vi "ccd_triggeredacquire_bkup.vi"() -> ()   [LabVIEW 2009]
panel:
  out "output path":path
  out "Y 3":dbl
  out "X 3":dbl
  out "Y 2":dbl
  out "X 2":dbl
  out "Image 2":T1(plugin-control)
  out "Image":T1(plugin-control)
  out "cameraName":dbl
  out "imageType":dbl
  out "trigger_number":dbl
  out "framenumber":dbl
  out "Y":dbl
  out "X":dbl
  in  "Trigger action":u32(ring)=1 items=["Disabled", "Trigger start of acquisition", "Trigger start of each buffer list", "Trigger each buffer", "Trigger each line (linescan)", "Trigger end of acquisition"]
  in  "Trigger Type":u32(ring) items=["External", "RTSI", "ISO In"]
  in  "Data frames / trigger":dbl=10.0
  in  "Video Frames / Data frame":dbl=15.0
  in  "GO":bool
  in  "stop":bool
  in  "Manual (up) or automatic (down)":bool
  in  "Or, read path automatically from:":path=path "\\\\Foghorn.bio.brandeis.edu\\remote"
  in  "Manual save directory":string
  in  "Manual save path":path
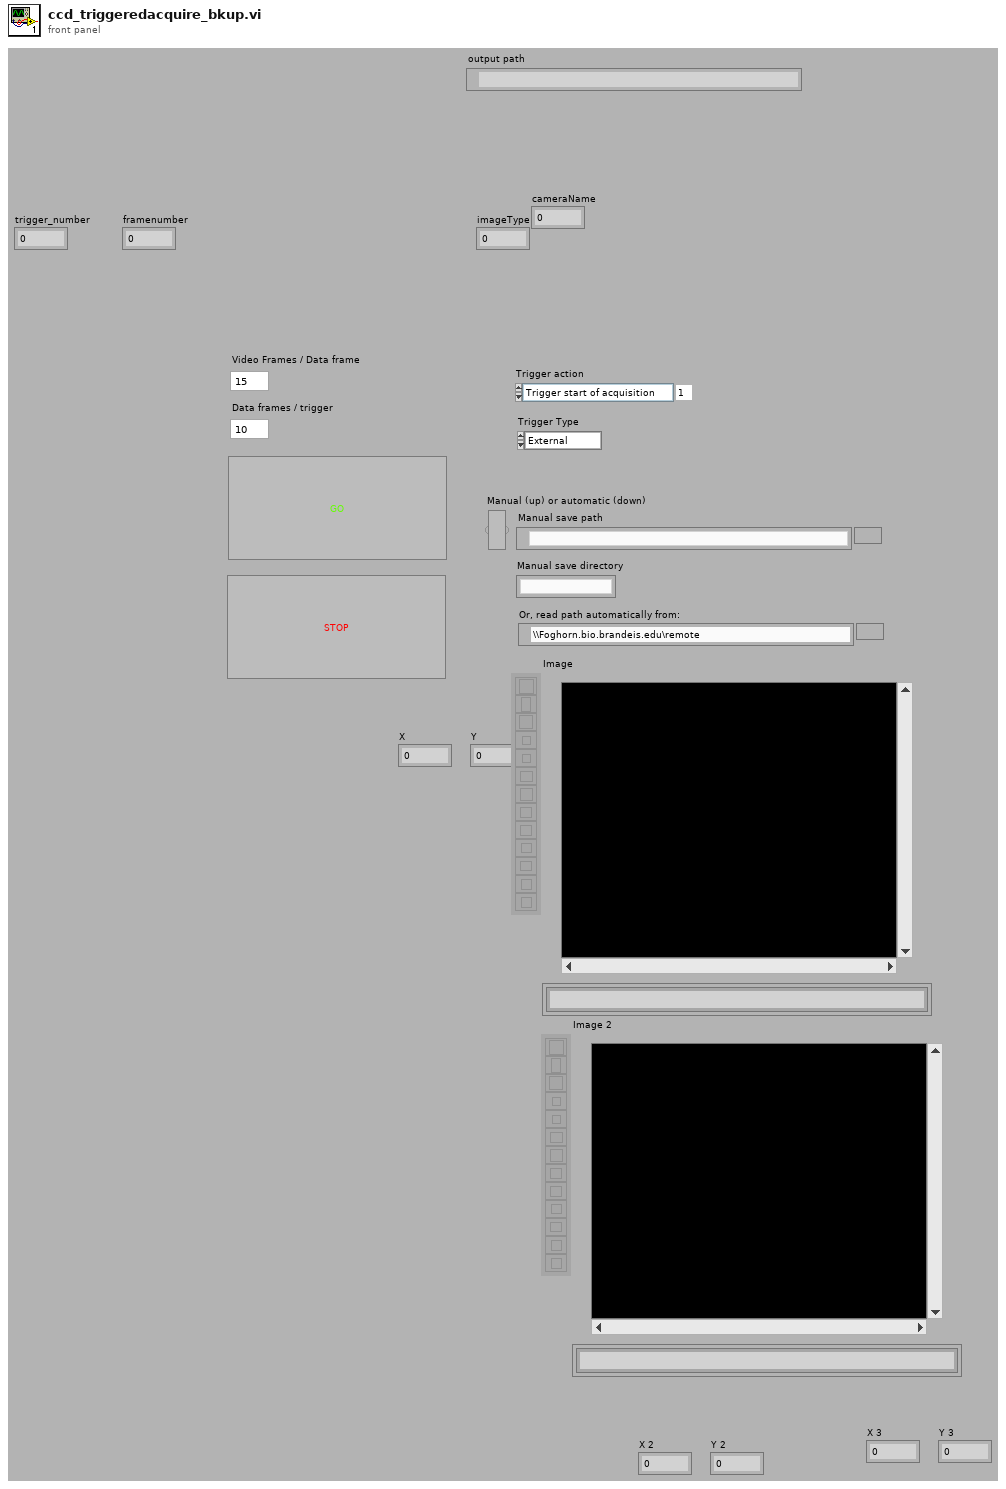
[diagram p1: front panel]
types:
  T1 = typedef "IMAQ Image.ctl" = refnum<image>
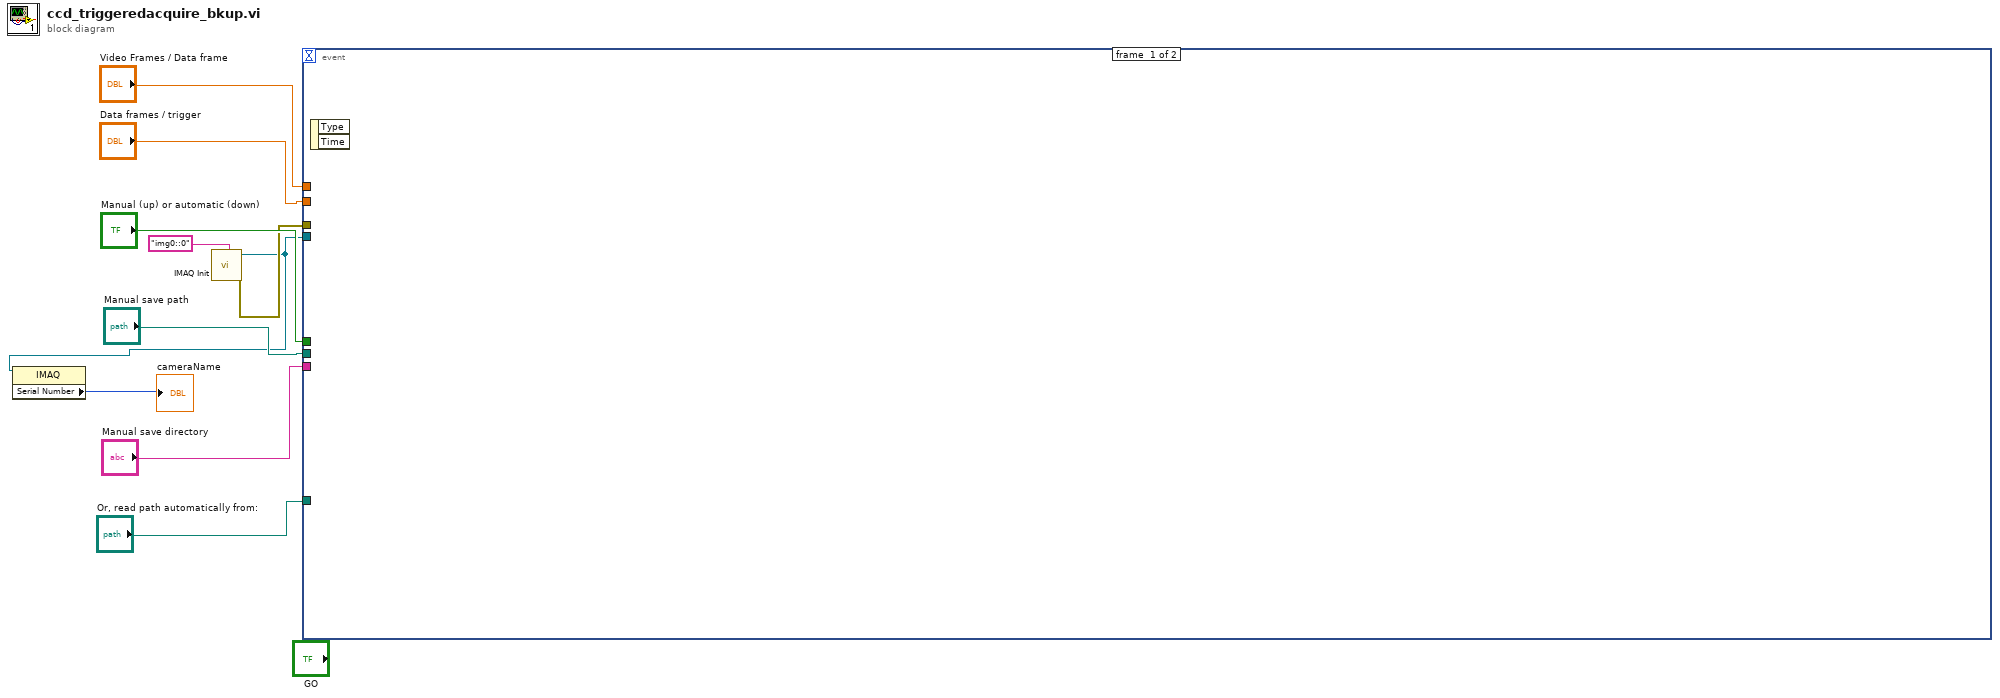
[diagram p0: block diagram]
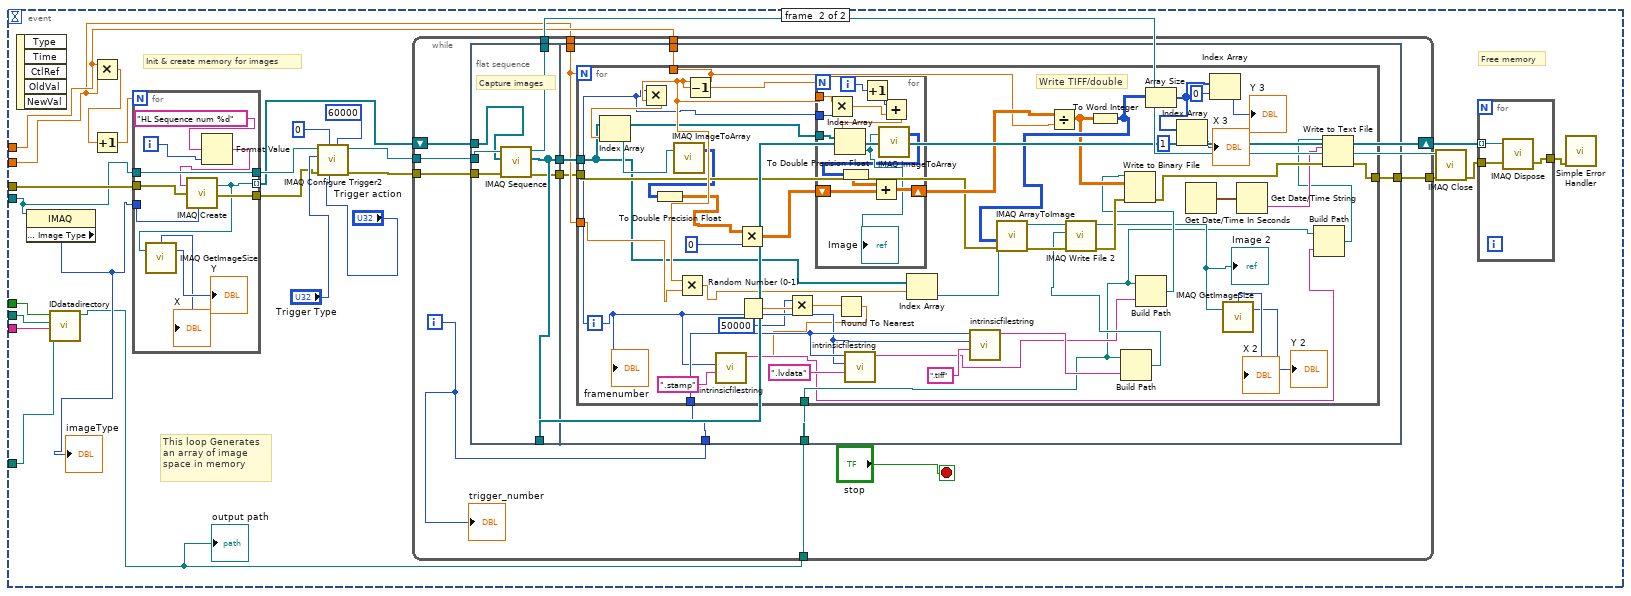
[diagram p2: hidden frame]
diagram:
  n1 = call <vilib>:"IMAQ Init.vi"("Interface Name"="img0::0") -> ("error out"=w4:errorcluster, "IMAQ Session Out"=w2:refnum<k11>)  [unwired: 9 in]
  n2 = property class="IMAQ"(reference=w2) -> ("Serial Number"=→"cameraName":u32)  [unwired: 1 in, 2 out]
  n3 = event shown="[1] \"GO\": Value Change" {
    selector: _ -> [_ _]
    dyn-events: _ -> [_ _]
    timeout: _ -> [_ _]
    tunnel: "Video Frames / Data frame" -> [_ w23]
    tunnel: "Data frames / trigger" -> [_ w22]
    tunnel: "Or, read path automatically from:" -> [_ w27]
    tunnel: "Manual save directory" -> [_ w26]
    tunnel: "Manual save path" -> [_ w25]
    tunnel: "Manual (up) or automatic (down)" -> [_ w24]
    tunnel: w4 -> [_ w15]
    tunnel: w2 -> [_ w14]
    event #0 {
      n4 = event-data() -> ()  [unwired: 1 in, 2 out]
    }
    event #1 {
      # "Free memory"
      # "This loop Generates an array of image space in memory"
      # "Init & create memory for images"
      n5 = event-data() -> ()  [unwired: 1 in, 5 out]
      n6 = property class="IMAQ"(reference=w14) -> ("Image Parameters : Image Type"=w13:u32)  [unwired: 1 in, 2 out]
      "imageType" <- w13
      n7 = call "IDdatadirectory.vi"("Read path automatically from:"=w27, "Directory"=w26, "Save path"=w25, "Manual or automatic"=w24) -> ("Outputpath"=w11:path)  [unwired: 7 in]
      "output path" <- w11
      n8 = Multiply(x=w23, y=w22) -> (x*y=w21:dbl)
      n9 = Increment(x=w21) -> (x+1=w20:dbl)
      n10 = for {
        N: w20 -> [_]
        tunnel: [w134] -> w32
        tunnel: [w130] -> w19 mode=indexing
        tunnel: w15 -> [w133]
        tunnel: w14 -> [w132]
        tunnel: [w132] -> w33
        tunnel: w13 -> [w131]
        i -> [w126]
        n11 = Format Value(format string="HL Sequence num %d", value (0)=w126) -> (output string=w125:string)  [unwired: 1 in]
        n12 = call "IMAQ Create"("Image Name"=w125, "Image Type"=w131, "error in (no error)"=w133) -> ("New Image"=w130:T1, "error out"=w134:errorcluster)  [unwired: 2 in]
        n13 = call "IMAQ GetImageSize"("Image"=w130) -> ("Y Resolution"=→"Y":i32, "X Resolution"=→"X":i32)  [unwired: 3 in, 1 out]
      }
      n14 = call <vilib>:"IMAQ Configure Trigger2.vi"("Frame timeout (ms)"=u32 60000, "Trigger action"="Trigger action", "Trigger Polarity"=0, "error in (no error)"=w32, "Trigger Type"="Trigger Type", "IMAQ Session In"=w33) -> ("error out"=w30:errorcluster, "IMAQ Session Out"=w31:refnum<k11>)  [unwired: 4 in]
      n15 = while {
        tunnel: w31 -> [w52]
        tunnel: w30 -> [w51]
        shift-right: [w43] -> w18
        shift-left: w19 -> [w45]
        tunnel: [w49] -> w28
        tunnel: w11 -> [w48]
        tunnel: w23 -> [w47]
        tunnel: w22 -> [w46]
        tunnel: [w41] -> w17
        i -> [w40]
        stop <- "stop" stop-if-true
        n16 = flat-sequence {
          tunnel: w52 -> [w56]
          tunnel: w51 -> [w58]
          tunnel: [w54] -> w50
          tunnel: [w57] -> w49
          tunnel: w45 -> [w55]
          tunnel: [w54] -> w43
          tunnel: [w53] -> w42
          tunnel: w50 -> [w65]
          tunnel: w48 -> [w64]
          tunnel: w40 -> [w59]
          tunnel: w47 -> [w63]
          tunnel: w46 -> [w62]
          tunnel: w42 -> [w61]
          tunnel: [w60] -> w41
          frame #0 {
            # "Capture images"
            n17 = call <vilib>:"IMAQ Sequence.vi"("error in (no error)"=w58, "Images In"=w55, "IMAQ Session In"=w56) -> ("error out"=w53:errorcluster, "Images Out"=w54:T1[], "IMAQ Session Out"=w57:refnum<k11>)  [unwired: 6 in]
          }
          frame #1 {
            n18 = for {
              N: w62 -> [_]
              tunnel: w65 -> [w69]
              tunnel: w64 -> [w80]
              tunnel: w59 -> [w82]
              tunnel: w63 -> [w107]
              tunnel: w62 -> [w109]
              tunnel: w61 -> [w105]
              tunnel: [w78] -> w60
              i -> [w81]
              # "Write TIFF/double"
              n19 = Multiply(x=w81, y=w107) -> (x*y=w111:dbl)
              n20 = Index Array(array=w69, index=w111) -> (element=w112:T1)
              n21 = call "IMAQ ImageToArray"("Image"=w112) -> ("Image Pixels (I16)"=w95:i16[][])  [unwired: 3 in, 4 out]
              n22 = To Double Precision Float(number=w95) -> (double precision float=w68:dbl[][])
              n23 = Multiply(x=w107, y=w109) -> (x*y=w106:dbl)
              n24 = Decrement(x=w107) -> (x-1=w110:dbl)
              n25 = Multiply(x=w68, y=0) -> (x*y=w67:dbl[][])
              n26 = Random Number (0-1)() -> (number: 0 to 1=w73:dbl)
              n27 = Multiply(x=50000, y=w73) -> (x*y=w71:dbl)
              n28 = for {
                N: w110 -> [_]
                tunnel: w69 -> [w124]
                shift-right: [w121] -> w108
                shift-left: w67 -> [w122]
                tunnel: w107 -> [w119]
                tunnel: w81 -> [w118]
                i -> [w120]
                n29 = Multiply(x=w119, y=w118) -> (x*y=w116:dbl)
                n30 = Increment(x=w120) -> (x+1=w117:i32)
                n31 = Add(x=w117, y=w116) -> (x+y=w115:dbl)
                n32 = Index Array(array=w124, index=w115) -> (element=w114:T1)
                "Image" <- w114
                n33 = call "IMAQ ImageToArray"("Image"=w114) -> ("Image Pixels (I16)"=w113:i16[][])  [unwired: 3 in, 4 out]
                n34 = To Double Precision Float(number=w113) -> (double precision float=w123:dbl[][])
                n35 = Add(x=w123, y=w122) -> (x+y=w121:dbl[][])
              }
              n36 = Round To Nearest(number=w71) -> (nearest integer value=w70:dbl)
              n37 = call "intrinsicfilestring.vi"("Postfix"=".stamp", "Frame number"=w81, "Trigger number"=w70) -> ("Filestring"=w79:string)  [unwired: 8 in]
              n38 = call "intrinsicfilestring.vi"("Postfix"=".lvdata", "Frame number"=w81, "Trigger number"=w82) -> ("Filestring"=w86:string)  [unwired: 8 in]
              n39 = Index Array(array=w69, index=w106) -> (element=w91:T1)
              n40 = call "intrinsicfilestring.vi"("Postfix"=".tiff", "Frame number"=w81, "Trigger number"=w82) -> ("Filestring"=w93:string)  [unwired: 8 in]
              n41 = Divide(x=w108, y=w107) -> (x/y=w87:dbl[][])
              n42 = To Word Integer(number=w87) -> (16bit integer=w94:i16[][])
              n43 = call "IMAQ ArrayToImage"("error in (no error)"=w105, "Image Pixels (I16)"=w94, "Image"=w91) -> ("error out"=w104:errorcluster, "Image Out"=w103:T1)  [unwired: 7 in]
              n44 = Build Path(base path=w80, name or relative path=w93) -> (appended path=w90:path)
              n45 = call-poly "IMAQ Write File 2"("error in (no error)"=w104, "File Path"=w90, "Image"=w103) -> ("error out"=w88:errorcluster, "Image Out (duplicate)"=w84:T1)  [unwired: 7 in]
              "Image 2" <- w84
              n46 = Build Path(base path=w80, name or relative path=w86) -> (appended path=w85:path)
              n47 = Write to Binary File(file (use dialog)=w85, data=w87, error in=w88) -> (error out=w77:errorcluster)  [unwired: 3 in, 2 out]
              n48 = Array Size(array=w94) -> (size(s)=w99:i32[])
              n49 = Index Array(array=w99, index=1) -> (element=→"X 3":i32)
              n50 = Get Date/Time In Seconds() -> (seconds since 1Jan1904=w74:timestamp)
              n51 = Index Array(array=w99, index=0) -> (element=→"Y 3":i32)
              n52 = call "IMAQ GetImageSize"("Image"=w84) -> ("Y Resolution"=→"Y 2":i32, "X Resolution"=→"X 2":i32)  [unwired: 3 in, 1 out]
              n53 = Get Date/Time String(seconds (now)=w74) -> (time string=w76:string)  [unwired: 2 in, 1 out]
              n54 = Build Path(base path=w80, name or relative path=w79) -> (appended path=w75:path)
              n55 = Write to Text File(file (use dialog)=w75, text=w76, error in=w77) -> (error out=w78:errorcluster)  [unwired: 1 in, 2 out]
              "framenumber" <- w81
            }
          }
        }
        "trigger_number" <- w40
      }
      n56 = call <vilib>:"IMAQ Close.vi"("error in (no error)"=w17, "IMAQ Session In"=w28) -> ("error out"=w16:errorcluster)  [unwired: 9 in]
      n57 = for {
        tunnel: w18 -> [w39] mode=indexing
        tunnel: w16 -> [w38]
        tunnel: [w37] -> w29
        n58 = call "IMAQ Dispose"("Image"=w39, "error in (no error)"=w38) -> ("error out"=w37:errorcluster)  [unwired: 4 in]
      }
      n59 = call <vilib>:"Simple Error Handler.vi"("error in (no error)"=w29) -> ()  [unwired: 4 in, 5 out]
    }
  }
